vi "Initialize.vi"(6 "Default return":variant, 7 "writer buffer size":i32=4096, 8 "error in (no error)":errorcluster, 9 "writer url":string, 10 "reader name":string) -> (0 "error out":errorcluster, 3 "NetworkStreamWriter out":refnum<class "NetworkStreamReader.lvclass">)   [LabVIEW 2011, in "NetworkStreamReader.lvclass"]
doc: "This VI returns an instance of the NetworkStreamReader class. A NetworkStreamReader attempts to open a network stream with a writer endpoint. As with network streams, the writer url on the reader or the reader url on the writer must be given before the connection can be made. Note that until a connection is made, this VI will not return. It will, however, stop on a commanded e-stop from the top-level VI. This VI also launches a reader daemon which constantly adds information passed across the stream to an internal queue accessed by the Read method."
uses:
  NetworkStreamReader.lvclass
  NetworkStreamReader.lvclass/NetworkStreamReader.ctl
  ReaderDaemon.vi
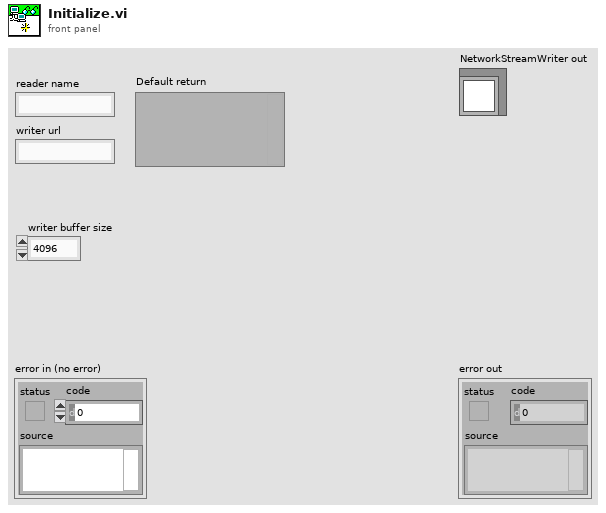
[diagram p1: front panel]
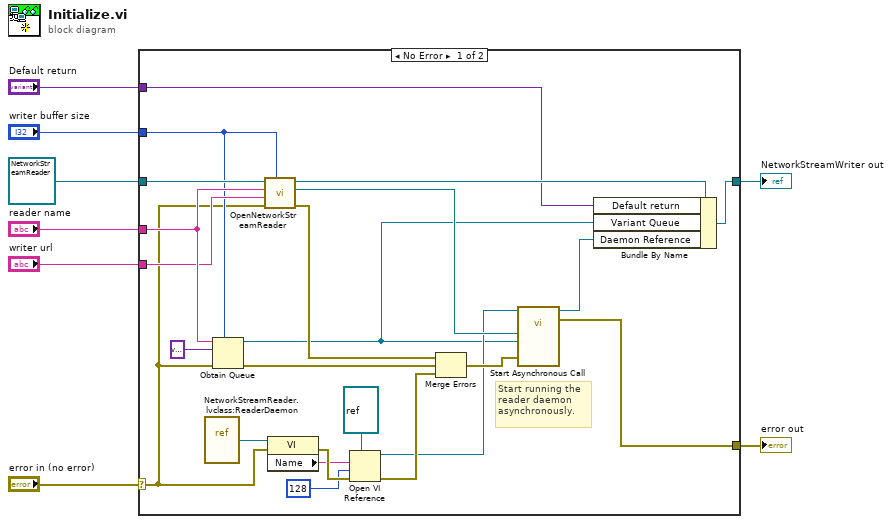
[diagram p0: block diagram]
diagram:
  n1 = case shown="No Error" "error in (no error)" {
    selector: "error in (no error)" -> [w17 w33]
    tunnel: [w11 w33] -> w7
    tunnel: [w25 w32] -> w6
    tunnel: refnum<class "NetworkStreamReader.lvclass"> refnum ("NetworkStreamWriter in") -> [w31 w32]
    tunnel: "reader name" -> [w30 _]
    tunnel: "writer url" -> [w29 _]
    tunnel: "writer buffer size" -> [w27 _]
    tunnel: "Default return" -> [w9 _]
    frame No Error {
      # "Start running the \nreader daemon\nasynchronously."
      n2 = vi-ref "NetworkStreamReader.lvclass:ReaderDaemon.vi"() -> (w18:refnum<vi>)
      n3 = Obtain Queue(max queue size (-1, unlimited)=w27, name (unnamed)=w30, element data type=variant, error in (no error)=w17) -> (queue out=w10:refnum<queue>, error out=w24:errorcluster)  [unwired: 1 in, 1 out]
      n4 = call "OpenNetworkStreamReader.vi"("reader buffer size"=w27, "error in (no error)"=w17, "writer url"=w29, "reader name"=w30, "NetworkStreamReader in"=w31) -> ("error out"=w23:errorcluster, "Reader Endpoint"=w14:refnum<k21>, "NetworkStreamReader out"=w26:refnum<class "NetworkStreamReader.lvclass">)  [unwired: 4 in]
      n5 = property class="VI"(reference=w18, error in=w17) -> (error out=w22:errorcluster, "Name"=w19:string)  [unwired: 1 out]
      n6 = Open VI Reference(type specifier VI Refnum (for type only)=refnum<vi> refnum, vi path=w19, options=128, error in (no error)=w22) -> (vi reference=w12:refnum<vi>, error out=w16:errorcluster)  [unwired: 2 in]
      n7 = Merge Errors(w23, w24, w16) -> (w15:errorcluster)
      n8 = call-by-ref "Start Asynchronous Call"(reference=w12, "error in (no error)"=w15, "Variant Queue"=w10, "Writer Endpoint"=w14) -> (reference out=w13:refnum<vi>, error out=w11:errorcluster)  [unwired: 10 in]
      n9 = Bundle By Name(cluster=w26, "Default return"=w9, "Variant Queue"=w10, "Daemon Reference"=w13) -> (w25:refnum<class "NetworkStreamReader.lvclass">)
    }
    frame Error {
    }
  }
  "error out" <- w7
  "NetworkStreamWriter out" <- w6
